vi "Find Chassis.vi"(6 "Map":map{string, T1}(c390), 11 "Hardware Type":T2) -> (2 "Chassis Info":T1[](array[typedef]), 3 "Has Chassis":bool)   [LabVIEW 2023, in "Volatus.lvlib" / "Hardware Info Module.lvclass"]
uses:
  Hardware Info Module.lvclass
  HW Info.ctl
  Hardware Type.ctl
  Hardware Info Module.lvclass/Hardware Info Module.ctl
  Volatus.lvlib
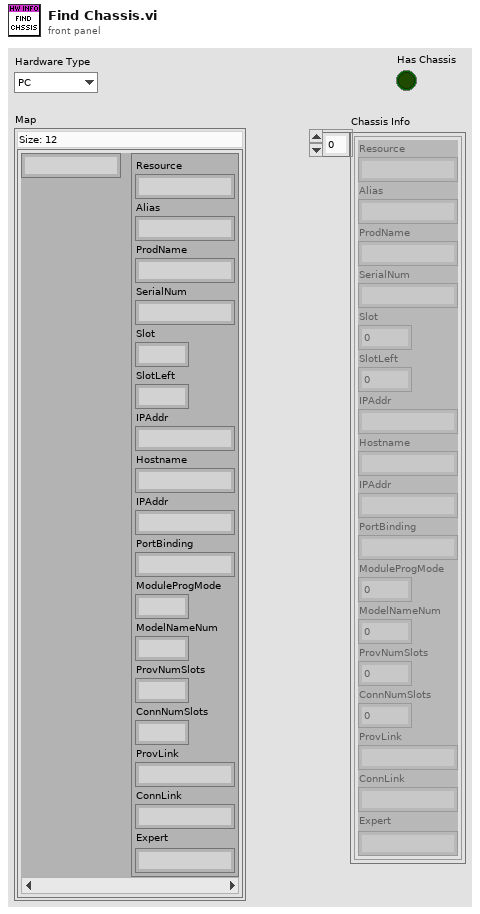
[diagram p1: front panel]
types:
  T1 = typedef "Volatus.lvlib/Hardware Info Module.lvclass/HW Info.ctl" = cluster{"Resource":string, "Alias":string, "ProdName":string, "SerialNum":string, "Slot":i32, "SlotLeft":u32, "IPAddr":string, "Hostname":string, "IPAddr":string, "PortBinding":string, "ModuleProgMode":u32, "ModelNameNum":u32, "ProvNumSlots":i32, "ConnNumSlots":i32, "ProvLink":string, "ConnLink":string, "Expert":string}
  T2 = typedef "Volatus.lvlib/Hardware Type.ctl" = enum16{"PC", "cRIO", "PXI"}
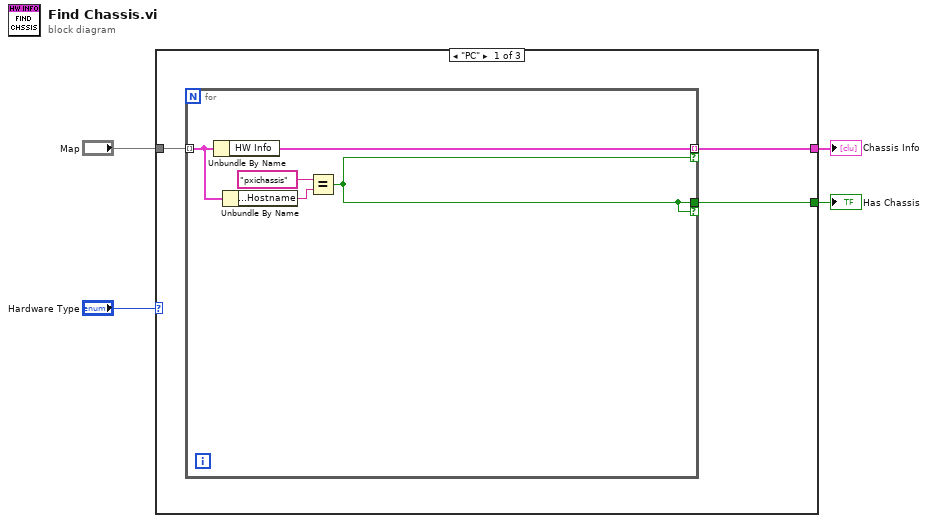
[diagram p0: block diagram]
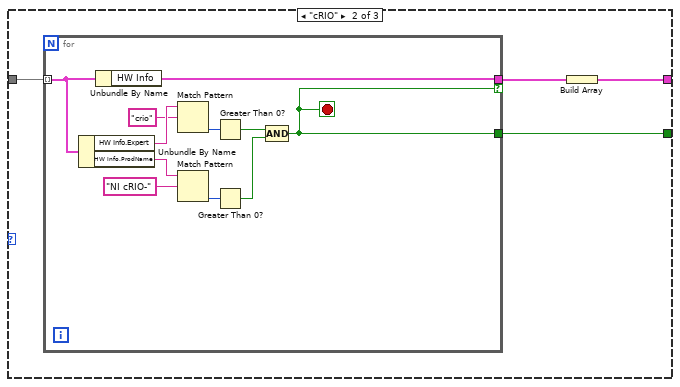
[diagram p2: hidden frame]
diagram:
  n1 = case shown="\"PC\"" "Hardware Type" {
    tunnel: [w5 w14 _] -> w3
    tunnel: "Map" -> [w7 w16 _]
    tunnel: [w6 w13 _] -> w1
    frame "PC" {
      n2 = for {
        tunnel: w7 -> [w12] mode=indexing
        tunnel: [w9] -> w6 mode=indexing if=w8
        tunnel: [w8] -> w5 if=w8
        n3 = Unbundle By Name(w12) -> ("HW Info"=w9:T1)
        n4 = Unbundle By Name(w12) -> ("HW Info.Hostname"=w11:string)
        n5 = Equal?(x="pxichassis", y=w11) -> (x = y?=w8:bool)
      }
    }
    frame "cRIO" {
      n6 = for {
        tunnel: w16 -> [w19] mode=indexing
        tunnel: [w18] -> w15 if=w17
        tunnel: [w17] -> w14
        stop <- w17 stop-if-true
        n7 = Unbundle By Name(w19) -> ("HW Info.Expert"=w27:string, "HW Info.ProdName"=w25:string)
        n8 = Unbundle By Name(w19) -> ("HW Info"=w18:T1)
        n9 = Match Pattern(string=w27, regular expression="crio") -> (offset past match=w22:i32)  [unwired: 1 in, 3 out]
        n10 = Match Pattern(string=w25, regular expression="NI cRIO-") -> (offset past match=w23:i32)  [unwired: 1 in, 3 out]
        n11 = Greater Than 0?(x=w22) -> (x > 0?=w21:bool)
        n12 = Greater Than 0?(x=w23) -> (x > 0?=w20:bool)
        n13 = Compound Arithmetic op=AND(w21, w20) -> (w17:bool)
      }
      n14 = Build Array(w15) -> (w13:T1[])
    }
    frame "PXI" {
    }
  }
  "Has Chassis" <- w3
  "Chassis Info" <- w1
